vi "Set Routing Channel Name.vi"(8 "error in":errorcluster, 10 "routing channel name":string, 11 "routing channel in":T1 format="%.0x") -> (0 "error out":errorcluster, 3 "routing channel out":T1 format="%.0x")   [LabVIEW 2019, in "Routing and Faulting Scripting.lvlib"]
doc: "Sets the name for the routing channel."
uses:
  Routing and Faulting Scripting.lvlib
  <vilib>/NI VeriStand/Custom Device API/Custom Device Item Ref.ctl
  <vilib>/NI VeriStand/Custom Device API/Custom Device API.lvlib
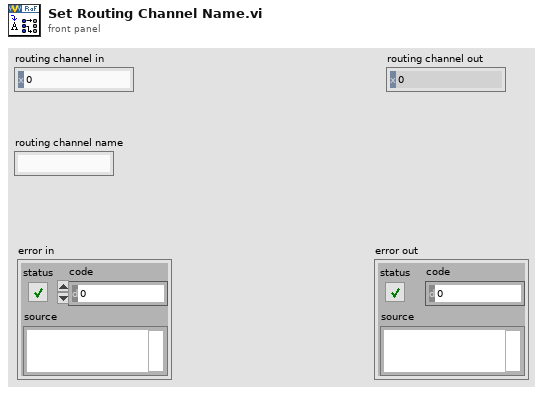
[diagram p1: front panel]
types:
  T1 = typedef "Custom Device API.lvlib/Custom Device Item Ref.ctl" = u64
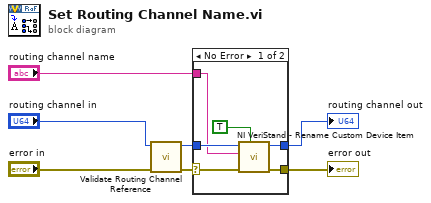
[diagram p0: block diagram]
diagram:
  n1 = call "Validate Routing Channel Reference.vi"("error in"="error in", "routing channel in"="routing channel in") -> ("error out"=w3:errorcluster, "routing channel out"=w1:T1)  [unwired: 8 in]
  n2 = case shown="No Error" w3 {
    selector: w3 -> [w9 w15]
    tunnel: [w11 w15] -> w7
    tunnel: [w12 w14] -> w6
    tunnel: w1 -> [w13 w14]
    tunnel: "routing channel name" -> [w10 _]
    frame No Error {
      n3 = call <vilib>:"NI VeriStand - Rename Custom Device Item.vi"("Force Rename (F)"=TRUE, "error in (no error)"=w9, "New Name"=w10, "Item Ref in"=w13) -> ("error out"=w11:errorcluster, "Item Ref out"=w12:T1)  [unwired: 5 in, 1 out]
    }
    frame Error {
    }
  }
  "error out" <- w7
  "routing channel out" <- w6
